vi "Digitizer Configure 2.vi"(7 "error in":errorcluster, 10 "Channel Parameters In":T1={"Channel Name"="0", "Number of Records"=0, "Reference Position"=0.0, "Minimum Record Length"=0, "Minimum Sample Rate"=0.0, "Maximum Input Frequency"=0.0, "Enforce Realtime"=FALSE, "Vertical Coupling"=enum."AC", "Probe Attenuation"=0.0, "Vertical Range (V)"=0.0, "Vertical Offset"=0.0, "Trigger Level"=0.0, "Trigger Type"=enum."Edge", "Trigger Source"=enum."Immediate", "Trigger Slope"=enum."Positive", "Digitizer 1 Used?"=FALSE, "Digitizer 1 Channels"="", "Digitizer 1 Reference"="", "Digitizer 1 Gain Multiplier"=nan, "Digitizer 2 Used?"=FALSE, "Digitizer 2 Channels"="", "Digitizer 2 Reference"="", "Session References"=[]}) -> (0 "error out":errorcluster, 3 "Channel Parameters Out":T1={"Channel Name"="0", "Number of Records"=0, "Reference Position"=0.0, "Minimum Record Length"=0, "Minimum Sample Rate"=0.0, "Maximum Input Frequency"=0.0, "Enforce Realtime"=FALSE, "Vertical Coupling"=enum."AC", "Probe Attenuation"=0.0, "Vertical Range (V)"=0.0, "Vertical Offset"=0.0, "Trigger Level"=0.0, "Trigger Type"=enum."Edge", "Trigger Source"=enum."Immediate", "Trigger Slope"=enum."Positive", "Digitizer 1 Used?"=FALSE, "Digitizer 1 Channels"="", "Digitizer 1 Reference"="", "Digitizer 1 Gain Multiplier"=nan, "Digitizer 2 Used?"=FALSE, "Digitizer 2 Channels"="", "Digitizer 2 Reference"="", "Session References"=[]})   [LabVIEW 2010]
uses:
  Typedef-Channel Parameters.ctl
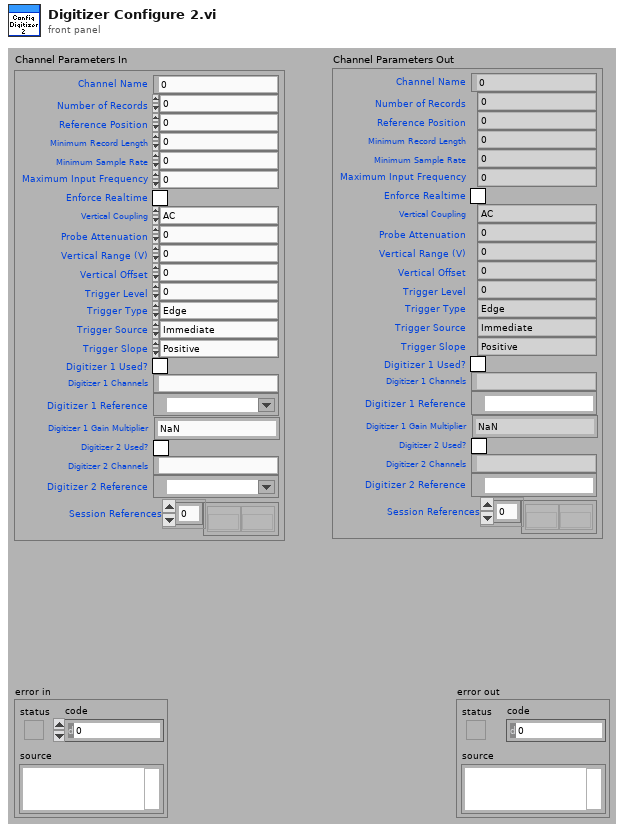
[diagram p1: front panel]
types:
  T1 = typedef "Typedef-Channel Parameters.ctl" = cluster{"Channel Name":string, "Number of Records":i32, "Reference Position":dbl, "Minimum Record Length":i32, "Minimum Sample Rate":dbl, "Maximum Input Frequency":dbl, "Enforce Realtime":bool, "Vertical Coupling":enum16{"AC", "DC", "Ground"}, "Probe Attenuation":dbl, "Vertical Range (V)":dbl, "Vertical Offset":dbl, "Trigger Level":dbl, "Trigger Type":enum16{"Edge", "Digital", "Immediate"}, "Trigger Source":enum16{"Immediate", "Channel 0", "Channel 1", "Channel 2", "Channel 3", "Channel 4", "Channel 5", "Channel 6", "Channel 7", "Extermal TRIG", "Software Trigger", "RTSI 0", "RTSI 1", "RTSI 2", "RTSI 3", "RTSI 4", "RTSI 5", "RTSI 6", "PF 0", "PF 1", "PF 2", "PXI Star Trigger"}, "Trigger Slope":enum16{"Positive", "Negative"}, "Digitizer 1 Used?":bool, "Digitizer 1 Channels":string, "Digitizer 1 Reference":refnum<k15>, "Digitizer 1 Gain Multiplier":dbl, "Digitizer 2 Used?":bool, "Digitizer 2 Channels":string, "Digitizer 2 Reference":refnum<k15>, "Session References":refnum<k20>[]}
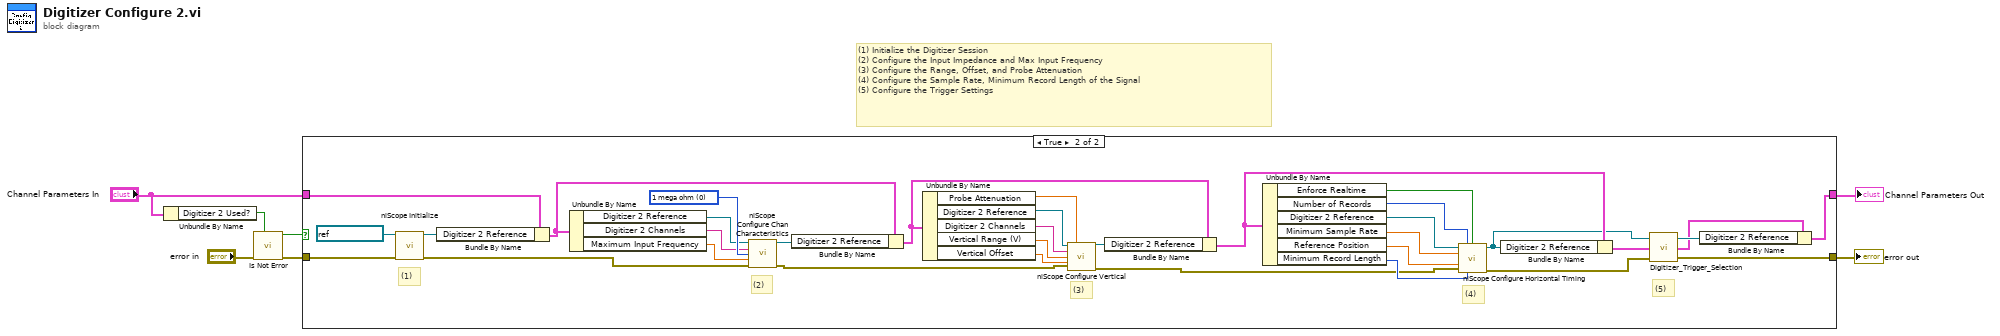
[diagram p0: block diagram]
diagram:
  # "(1) Initialize the Digitizer Session\n(2) Configure the Input Impedance and Max Input Frequency\n(3) Configure the Range, Offset, and Probe Attenuation\n(4) Configure the Sample Rate, Minimum Record Length of the Signal\n(5) Configure the Trigger Settings"
  n1 = Unbundle By Name("Channel Parameters In") -> ("Digitizer 2 Used?"=w2:bool)
  n2 = call "Is Not Error.vi"("enable (T)"=w2, "error in"="error in") -> ("error out"=w4:errorcluster, "!error"=w1:bool)  [unwired: 4 in, 1 out]
  n3 = case shown="True" w1 {
    tunnel: [w9 w41] -> w7
    tunnel: "Channel Parameters In" -> [w8 w40]
    tunnel: w4 -> [w9 w42]
    tunnel: [w8 w35] -> w5
    frame False {
    }
    frame True {
      w34 = u32 0 items=["1 mega ohm"=0, "50 ohms"=2] ("input impedance")
      # "(3)"
      # "(4)"
      # "(2)"
      # "(5)"
      # "(1)"
      n4 = call <instrlib>:"niScope Initialize.vi"("resource name"=refnum<k15> "PXI1Slot4", "error in"=w42) -> ("instrument handle"=w39:refnum<k15>, "error out"=w31:errorcluster)  [unwired: 12 in]
      n5 = Bundle By Name(cluster=w40, "Digitizer 2 Reference"=w39) -> (w29:T1)
      n6 = Unbundle By Name(w29) -> ("Digitizer 2 Reference"=w33:refnum<k15>, "Digitizer 2 Channels"=w32:string, "Maximum Input Frequency"=w28:dbl)
      n7 = call <instrlib>:"niScope Configure Chan Characteristics.vi"("instrument handle"=w33, "channels"=w32, "input impedance"=w34, "maximum input frequency"=w28, "error in"=w31) -> ("instrument handle out"=w30:refnum<k15>, "error out"=w15:errorcluster)  [unwired: 9 in]
      n8 = Bundle By Name(cluster=w29, "Digitizer 2 Reference"=w30) -> (w13:T1)
      n9 = Unbundle By Name(w13) -> ("Probe Attenuation"=w17:dbl, "Digitizer 2 Reference"=w18:refnum<k15>, "Digitizer 2 Channels"=w19:string, "Vertical Range (V)"=w20:dbl, "Vertical Offset"=w16:dbl)
      n10 = call <instrlib>:"niScope Configure Vertical.vi"("instrument handle"=w18, "probe attenuation"=w17, "channels"=w19, "vertical range"=w20, "vertical offset"=w16, "error in"=w15) -> ("instrument handle out"=w14:refnum<k15>, "error out"=w10:errorcluster)  [unwired: 8 in]
      n11 = Bundle By Name(cluster=w13, "Digitizer 2 Reference"=w14) -> (w12:T1)
      n12 = Unbundle By Name(w12) -> ("Enforce Realtime"=w22:bool, "Number of Records"=w23:i32, "Digitizer 2 Reference"=w27:refnum<k15>, "Minimum Sample Rate"=w26:dbl, "Reference Position"=w25:dbl, "Minimum Record Length"=w24:i32)
      n13 = call <instrlib>:"niScope Configure Horizontal Timing.vi"("instrument handle"=w27, "number of records"=w23, "enforce realtime"=w22, "min sample rate"=w26, "reference position"=w25, "error in"=w10, "min record length"=w24) -> ("instrument handle out"=w11:refnum<k15>, "error out"=w21:errorcluster)  [unwired: 7 in]
      n14 = Bundle By Name(cluster=w12, "Digitizer 2 Reference"=w11) -> (w38:T1)
      n15 = call "Digitizer_Trigger_Selection.vi"("Error In"=w21, "Channel Parameters In"=w38, "instrument handle in"=w11) -> ("error out"=w41:errorcluster, "Channel Parameters Out"=w36:T1, "instrument handle out"=w37:refnum<k15>)
      n16 = Bundle By Name(cluster=w36, "Digitizer 2 Reference"=w37) -> (w35:T1)
    }
  }
  "error out" <- w7
  "Channel Parameters Out" <- w5
